vi "ReadBytesAtPort.vi"(8 "Error In":errorcluster, 11 "Omega CSi32 In":refnum<visa-resource-name>) -> (0 "Error Out":errorcluster, 2 "Read Buffer":string, 3 "Omega CSi32 Out":refnum<visa-resource-name>)   [LabVIEW 2012, in "Omega-CSi32.lvlib"]
uses:
  Omega-CSi32.lvlib
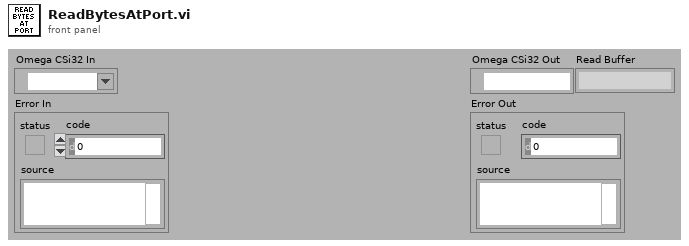
[diagram p1: front panel]
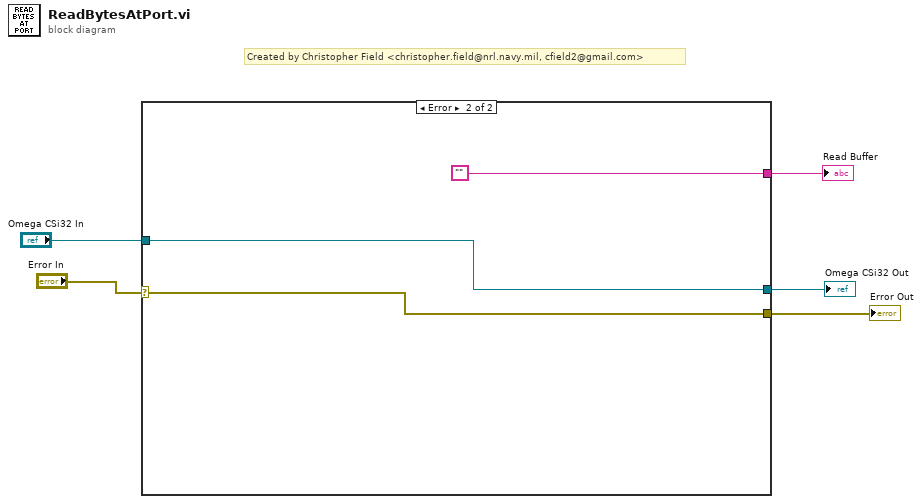
[diagram p0: block diagram]
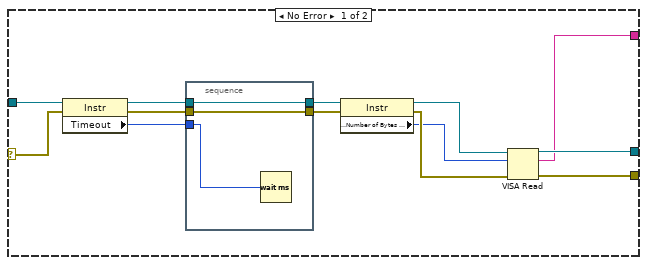
[diagram p2: hidden frame]
diagram:
  # "Created by Christopher Field <christopher.field@nrl.navy.mil, cfield2@gmail.com>"
  n1 = case shown="Error" "Error In" {
    selector: "Error In" -> [w6 w23]
    tunnel: [w15 w24] -> w5
    tunnel: [w14 w23] -> w4
    tunnel: [w13 ""] -> w3
    tunnel: "Omega CSi32 In" -> [w12 w24]
    frame No Error {
      n2 = property class="Instr"(reference=w12, error in=w6) -> (reference out=w11:refnum<visa-resource-name>, error out=w8:errorcluster, "Timeout"=w9:u32)
      n3 = stacked-sequence {
        tunnel: w11 -> [w21]
        tunnel: [w21] -> w10
        tunnel: w9 -> [w20]
        tunnel: w8 -> [w19]
        tunnel: [w19] -> w7
        frame #0 {
          n4 = Wait (ms)(milliseconds to wait=w20) -> ()  [unwired: 1 out]
        }
      }
      n5 = property class="Instr"(reference=w10, error in=w7) -> (reference out=w18:refnum<visa-resource-name>, error out=w17:errorcluster, "Serial Settings:Number of Bytes at Serial Port"=w16:u32)
      n6 = VISA Read(VISA resource name=w18, byte count=w16, error in (no error)=w17) -> (VISA resource name out=w15:refnum<visa-resource-name>, read buffer=w13:string, error out=w14:errorcluster)  [unwired: 1 out]
    }
    frame Error {
    }
  }
  "Omega CSi32 Out" <- w5
  "Error Out" <- w4
  "Read Buffer" <- w3
